vi "Write Image Graph.vi"(8 "error in (no error)":errorcluster, 10 "file path":string, 11 "Display Image in":refnum<class "Display Image.lvclass">) -> (0 "error out":errorcluster, 3 "Display Image out":refnum<class "Display Image.lvclass">)   [LabVIEW 2018, in "Display Image.lvclass"]
doc: "Este VI possui como entrada o caminho do arquivo FITS a ser lido, retornando o array da imagem do arquivo."
uses:
  Display Image.lvclass
  Display Image.lvclass/Display Image.ctl
  <userlib>/gfitsio/gfitsio-read-image-subset-i16-2d.vi
  <userlib>/gfitsio/gfitsio.lvlib
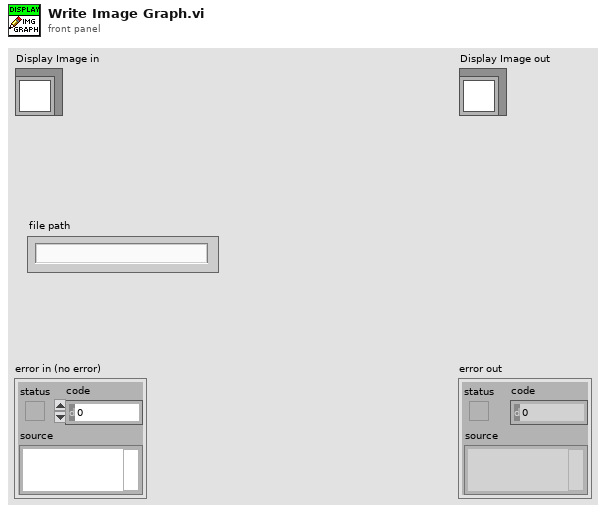
[diagram p1: front panel]
types:
  T1 = enum16{"open", "open or create", "create or replace", "create", "open (read only)"}
  T2 = typedef "gfitsio.lvlib/gfitsio-refnum.ctl" = refnum<k1>
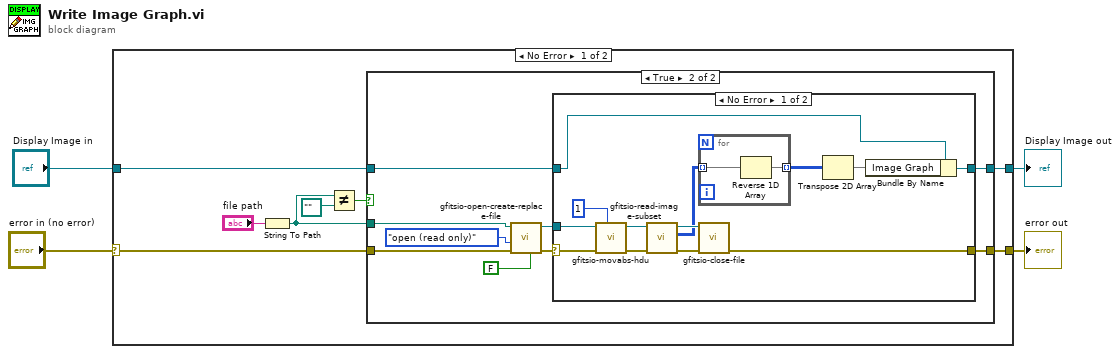
[diagram p0: block diagram]
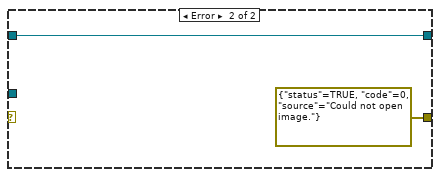
[diagram p3: hidden frame]
diagram:
  n1 = case shown="No Error" "error in (no error)" {
    selector: "error in (no error)" -> [w12 w42]
    tunnel: [w11 w42] -> w1
    tunnel: [w10 w41] -> w2
    tunnel: "Display Image in" -> [w9 w41]
    frame No Error {
      n2 = String To Path(string="file path") -> (path=w6:path)
      n3 = Not Equal?(x=w6, y=path "") -> (x != y?=w8:bool)
      n4 = case shown="True" w8 {
        tunnel: w12 -> [w13 w23]
        tunnel: [w13 w22] -> w11
        tunnel: [w14 w20] -> w10
        tunnel: w9 -> [w14 w17]
        tunnel: w6 -> [_ w15]
        frame False {
        }
        frame True {
          n5 = call <userlib>:"gfitsio-open-create-replace-file.vi"("advisory dialog? (display:T)"=FALSE, "error in (no error)"=w23, "function (open)"=T1."open (read only)", "file path (dialog if empty)"=w15) -> ("error out"=w18:errorcluster, "gfits refnum"=w19:T2)  [unwired: 5 in, 1 out]
          n6 = case shown="No Error" w18 {
            selector: w18 -> [w24 _]
            tunnel: [w35 errorcluster {"status"=TRUE, "code"=0, "source"="Could not open image."} ("error out")] -> w22
            tunnel: w17 -> [w30 w40]
            tunnel: [w29 w40] -> w20
            tunnel: w19 -> [w27 _]
            frame No Error {
              n7 = call <userlib>:"gfitsio-movabs-hdu.vi"("hdunum"=1, "error in (no error)"=w24, "gfits refnum"=w27) -> ("error out"=w28:errorcluster, "dup gfits refnum"=w26:T2)  [unwired: 6 in, 1 out]
              n8 = call-poly <userlib>:"gfitsio-read-image-subset.vi"("error in (no error)"=w28, "gfits refnum"=w26) -> ("error out"=w36:errorcluster, "data"=w32:i16[][], "dup gfits refnum"=w34:T2)  [unwired: 6 in, 1 out]
              n9 = for {
                tunnel: [w38] -> w33 mode=indexing
                tunnel: w32 -> [w37] mode=indexing
                n10 = Reverse 1D Array(array=w37) -> (reversed array=w38:i16[])
              }
              n11 = call <userlib>:"gfitsio-close-file.vi"("error in (no error)"=w36, "gfits refnum"=w34) -> ("error out"=w35:errorcluster)  [unwired: 8 in, 1 out]
              n12 = Transpose 2D Array(2D array=w33) -> (transposed array=w31:i16[][])
              n13 = Bundle By Name(cluster=w30, "Image Graph"=w31) -> (w29:refnum<class "Display Image.lvclass">)
            }
            frame Error {
            }
          }
        }
      }
    }
    frame Error {
    }
  }
  "error out" <- w1
  "Display Image out" <- w2
